vi "ConfigPlots.vi"(5 "曲线自定义封存数组":refnum<vi>, 7 "Y轴手配":refnum<vi>, 8 "Y标尺总数":i32, 9 "曲线手配":refnum<vi>, 10 "已选信号列表":refnum<vi>) -> ()   [LabVIEW 2015]
uses:
  Ctrls/btnSeeOrNot.ctl
panel:
  out "txtYlink":string
  out "txtUnit":string
  out "txtCurves":string
  out "txtYVisable":string
  out "txtSignal":string
  out "txtRename":string
  out "txtYName":string
  out "txtYsn":string
  out "txtYSetupTitle":string caption="txtYSetup"
  out "txtCurvesSetup":string
  in  "取消并退出按钮":bool
  in  "保存曲线设置按钮":bool
  in  "曲线设置输入簇数组":T1(array[cluster]) {"关联Y轴" min=1 max=8 format="Y轴%d"; "曲线序号" format="曲线%d"}
  in  "曲线簇":T2={"曲线序号"=0, "SignalName"="", "SignalTag"="", "自定义名"="", "单位"="", "关联Y轴"=1} {"关联Y轴" min=1 max=8 format="Y轴%d"; "曲线序号" format="曲线%d"}
  in  "Y簇":T4
  in  "Y轴配置":T5(array[cluster])
  out "自动Y轴配置":cluster{"Y轴序号":u8, "Y轴名称":string, "可见性":bool}[](array[cluster])
  out "自动曲线配置":T1(array[cluster])
  in  "曲线配置簇":T2
  in  "Y轴配置簇":cluster{"Y轴序号":u8, "Y轴名称":string, "可见性":bool}
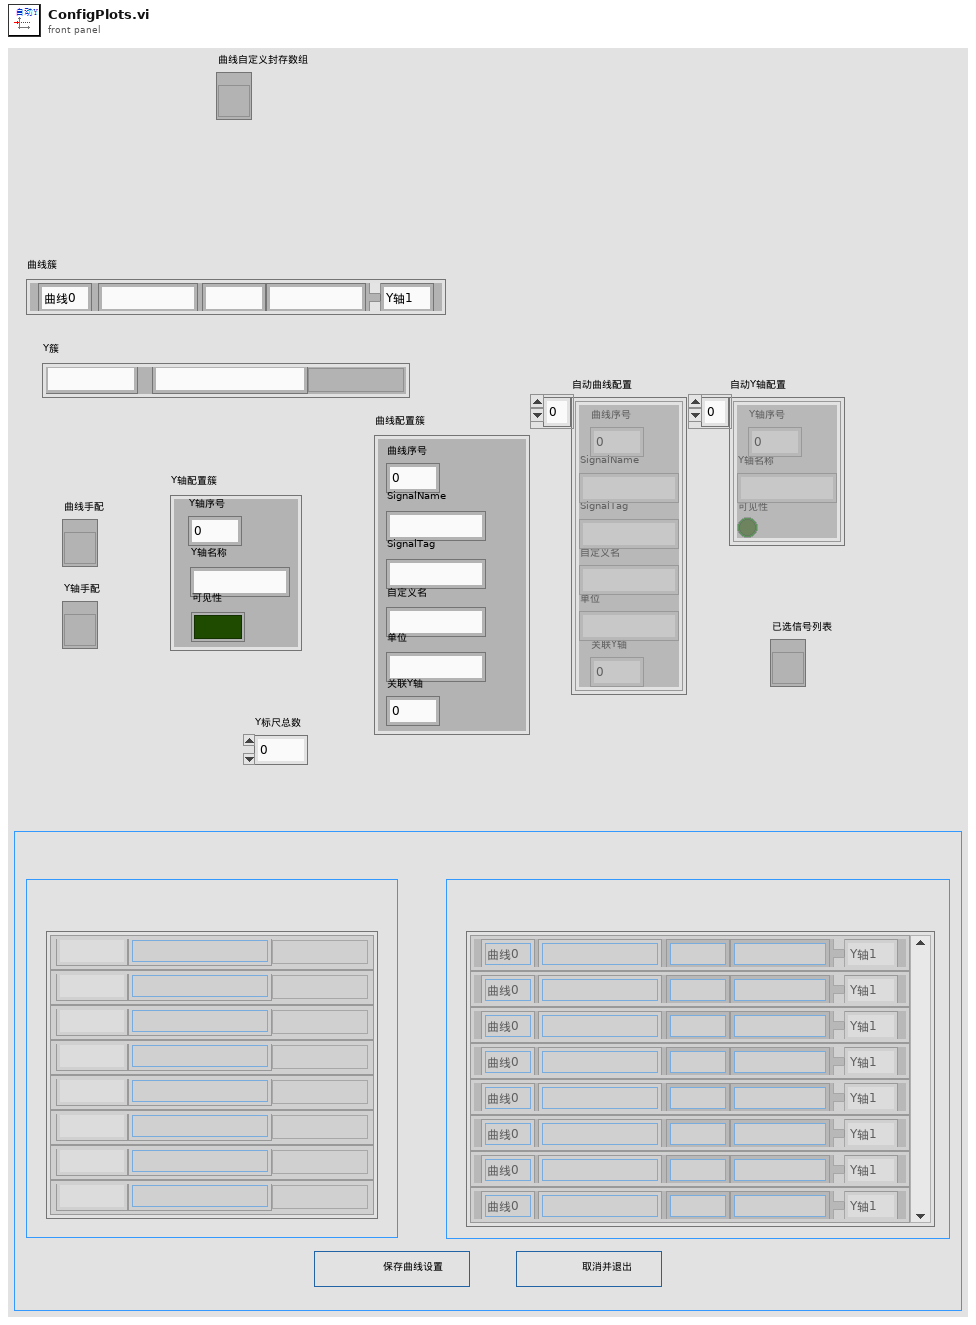
[diagram p1: front panel]
types:
  T1 = cluster{"曲线序号":u8, "SignalName":string, "SignalTag":string, "自定义名":string, "单位":string, "关联Y轴":u8}[]
  T2 = cluster{"曲线序号":u8, "SignalName":string, "SignalTag":string, "自定义名":string, "单位":string, "关联Y轴":u8}
  T3 = typedef "btnSeeOrNot.ctl" = bool
  T4 = cluster{"Y轴名称 2":string, "Y轴序号 2":string, "可见性":T3}
  T5 = cluster{"Y轴名称 2":string, "Y轴序号 2":string, "可见性":T3}[]
  T6 = typedef "可不可见.ctl" = bool
  T7 = cluster{"Y轴名称 2":string, "Y轴序号 2":string, "可见性":T6}
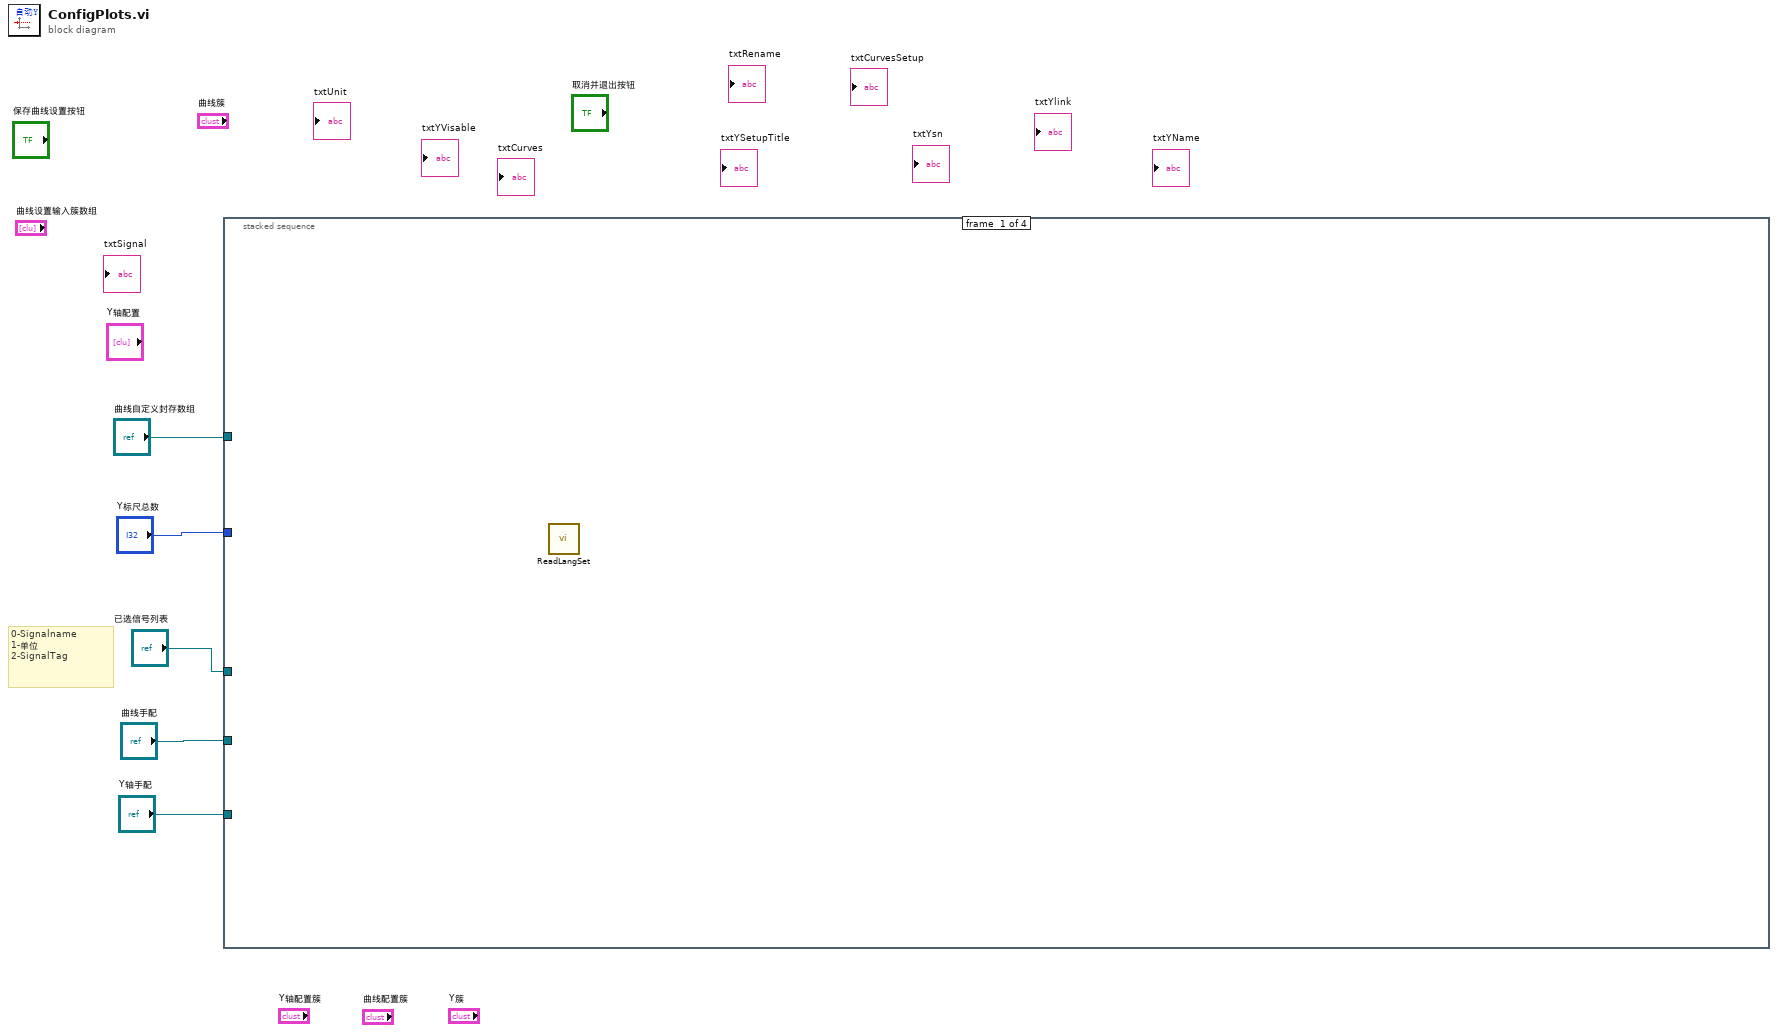
[diagram p0: block diagram]
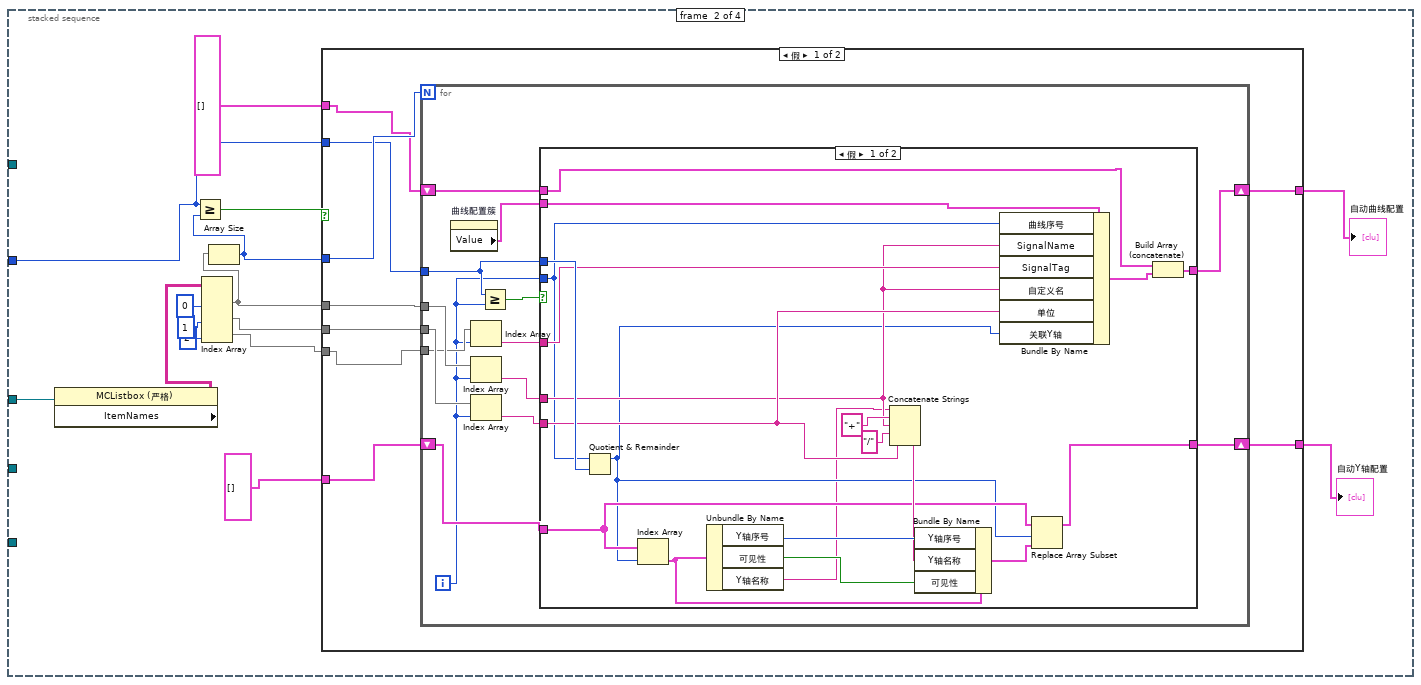
[diagram p2: hidden frame]
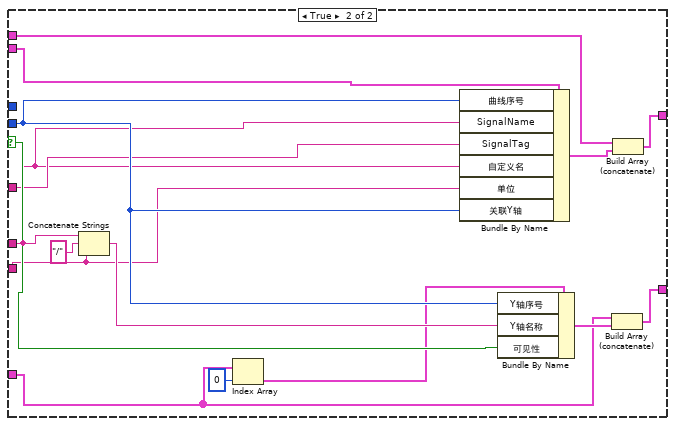
[diagram p3: hidden frame]
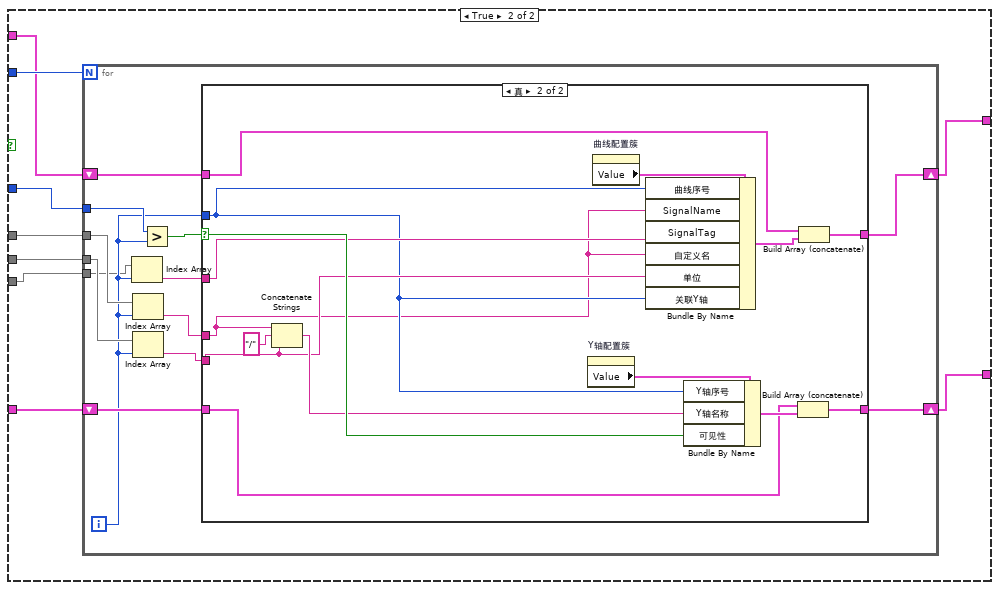
[diagram p4: hidden frame]
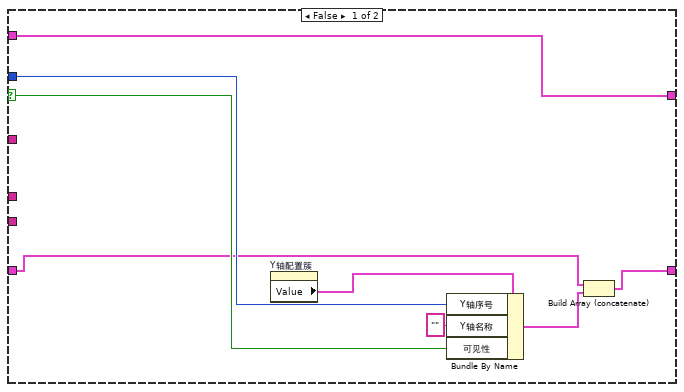
[diagram p5: hidden frame]
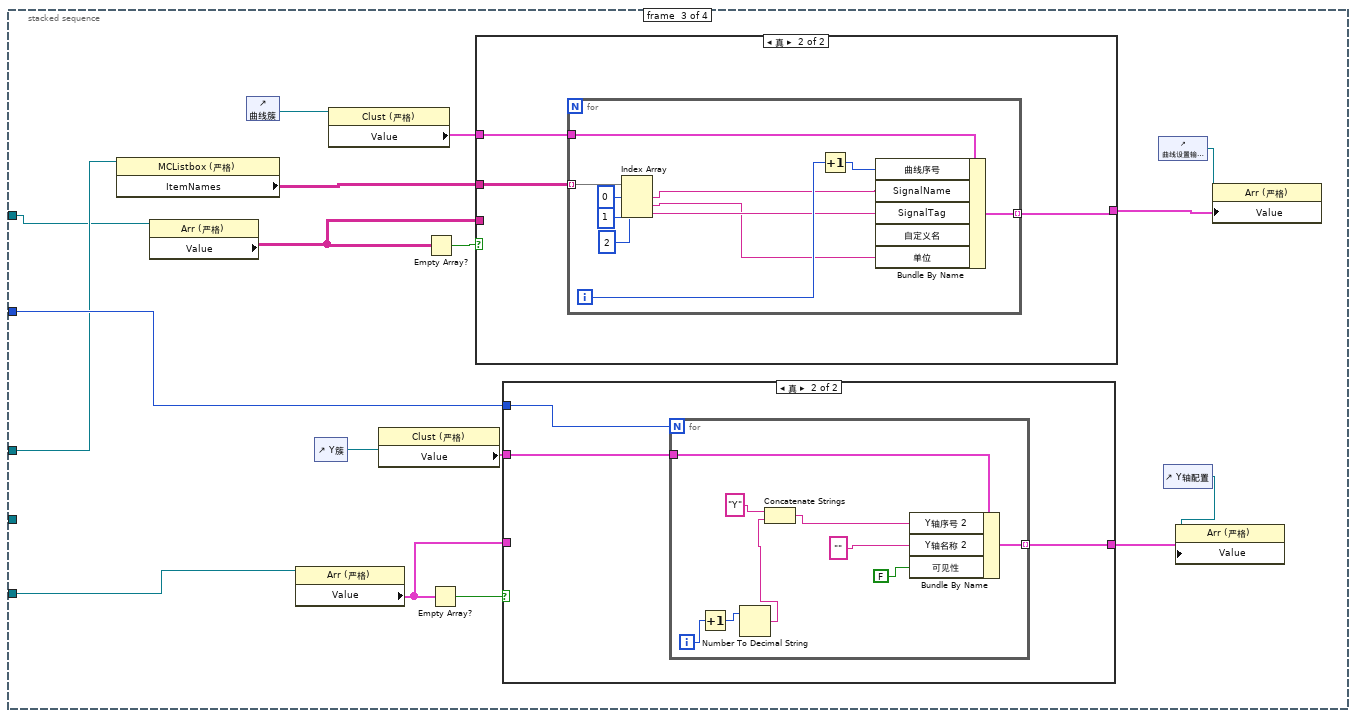
[diagram p6: hidden frame]
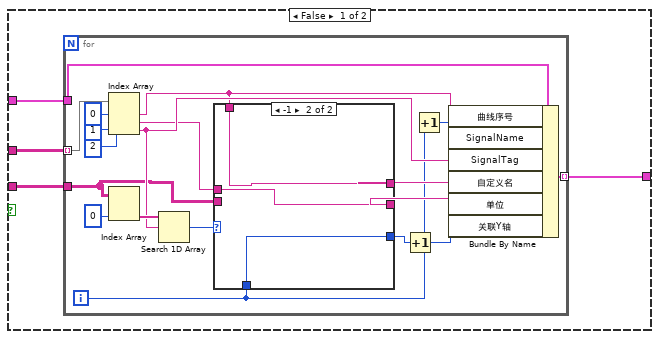
[diagram p7: hidden frame]
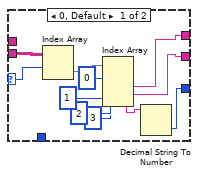
[diagram p8: hidden frame]
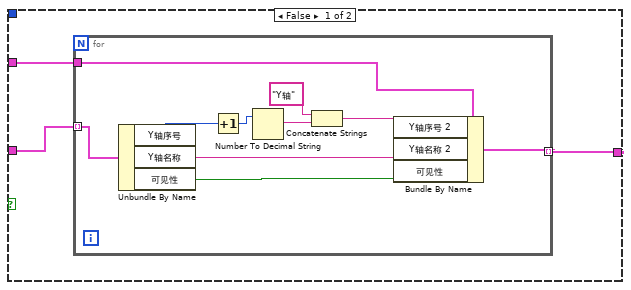
[diagram p9: hidden frame]
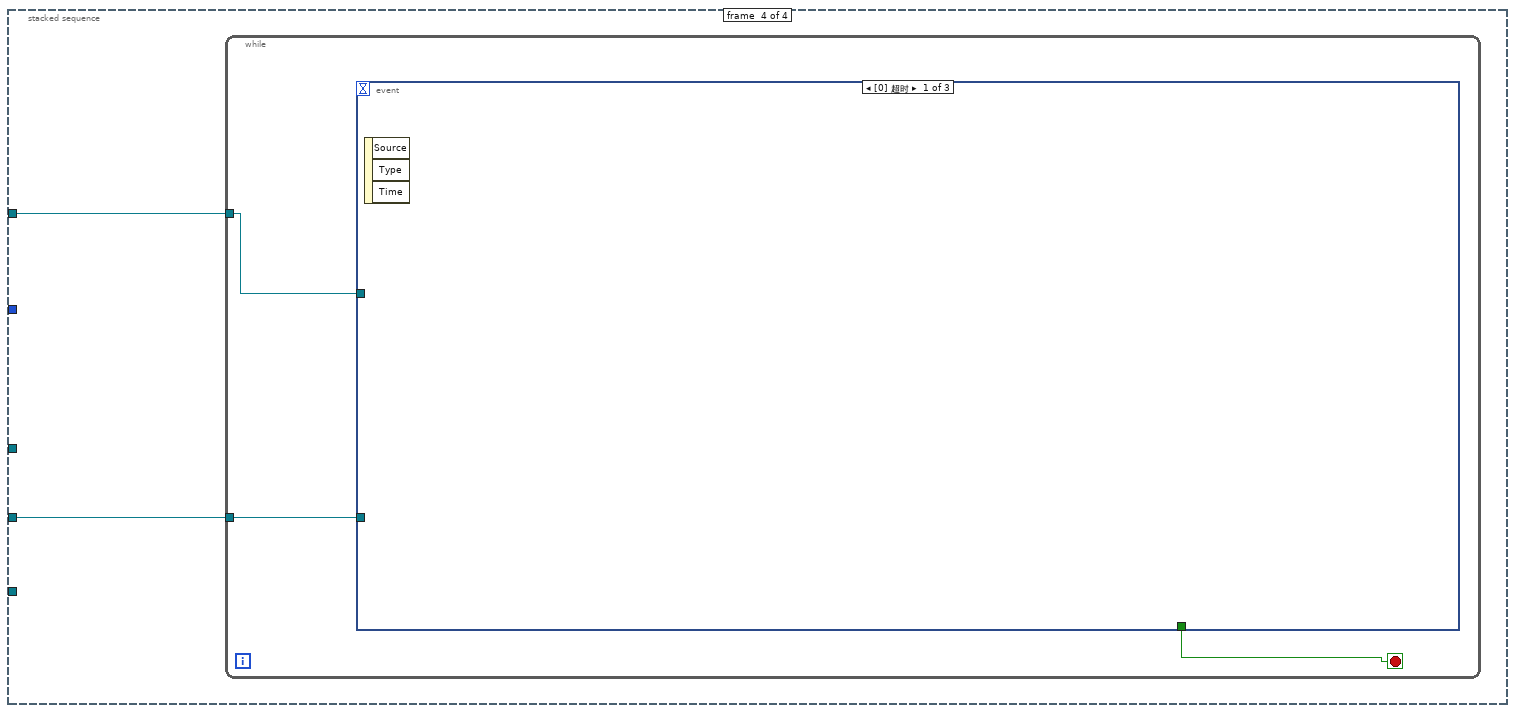
[diagram p10: hidden frame]
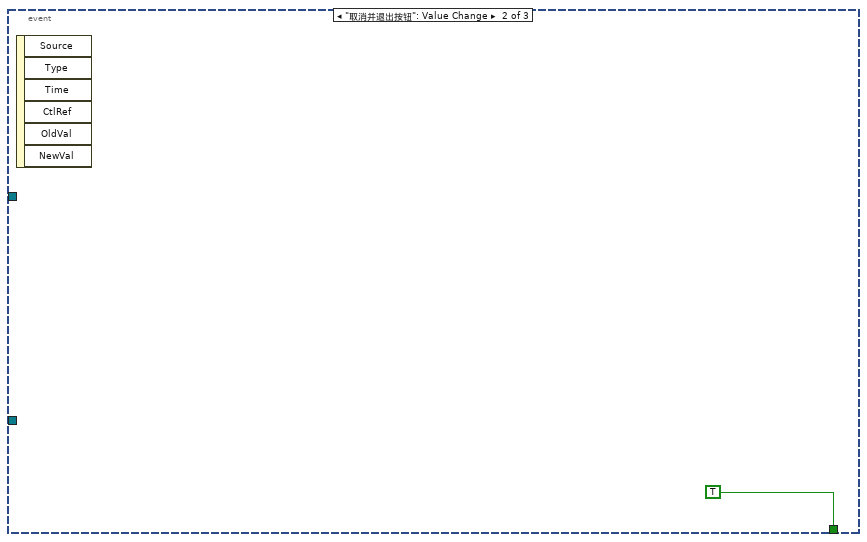
[diagram p11: hidden frame]
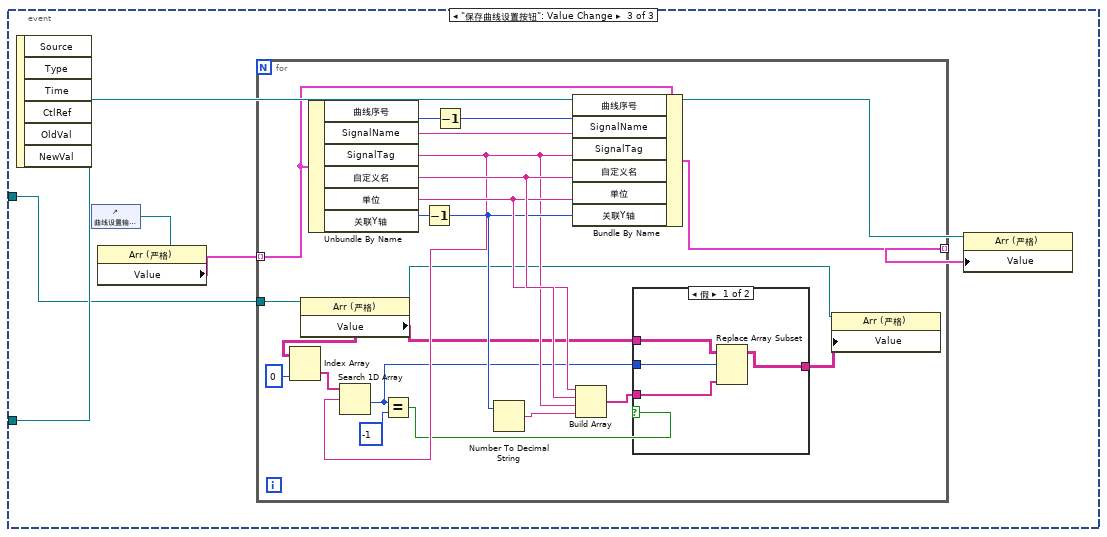
[diagram p12: hidden frame]
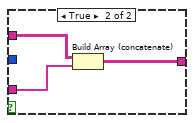
[diagram p13: hidden frame]
diagram:
  # "0-Signalname\n1-单位\n2-SignalTag"
  n1 = stacked-sequence {
    tunnel: "Y标尺总数" -> [_ w16 w134 _]
    tunnel: "已选信号列表" -> [_ w7 w127 _]
    tunnel: "曲线手配" -> [_ _ _ w219]
    tunnel: "Y轴手配" -> [_ _ w141 _]
    tunnel: "曲线自定义封存数组" -> [_ _ w125 w218]
    frame #0 {
      n2 = call "ReadLangSet.vi"() -> ()  [unwired: 11 in, 1 out]
    }
    frame #1 {
      n3 = property class="MCListbox (严格)"(reference=w7) -> ("ItemNames"=w6:string[][])  [unwired: 1 in, 2 out]
      n4 = Index Array(array=w6, index (col) #1=0 ("禁用的索引 (列)"), index (col) #2=1 ("索引 (列)"), index (col) #3=2 ("索引 (列)")) -> (element #1=w18:string[], element #2=w19:string[], element #3=w12:string[])  [unwired: 3 in]
      n5 = Array Size(array=w18) -> (size(s)=w20:i32)
      n6 = Greater Or Equal?(x=w16, y=w20) -> (x >= y?=w15:bool)
      n7 = case shown="假" w15 {
        tunnel: w16 -> [w26 w88]
        tunnel: w18 -> [w28 w87]
        tunnel: w19 -> [w29 w86]
        tunnel: w20 -> [w27 w85]
        tunnel: w12 -> [w24 w84]
        tunnel: cluster{"Y轴序号":u8, "Y轴名称":string, "可见性":bool}[] [] -> [w25 w83]
        tunnel: T1 [] -> [w23 w82]
        tunnel: [w22 w80] -> w8
        tunnel: [w21 w81] -> w9
        frame False {
          n8 = for {
            N: w27 -> [_]
            tunnel: w28 -> [w40]
            tunnel: w29 -> [w39]
            tunnel: w26 -> [w38]
            shift-right: [w37] -> w22
            shift-left: w25 -> [w36]
            tunnel: w24 -> [w35]
            shift-right: [w32] -> w21
            shift-left: w23 -> [w31]
            i -> [w34]
            n9 = property on="曲线配置簇" class="Clust (严格)"() -> ("Value"=w30:T2)  [unwired: 2 in, 2 out]
            n10 = Index Array(array=w35, index=w34) -> (element=w33:string)
            n11 = Index Array(array=w40, index=w34) -> (element=w42:string)
            n12 = Index Array(array=w39, index=w34) -> (element=w41:string)
            n13 = Greater Or Equal?(x=w38, y=w34) -> (x >= y?=w43:bool)
            n14 = case shown="假" w43 {
              selector: w43 -> [_ w75]
              tunnel: w34 -> [w56 w73]
              tunnel: w42 -> [w57 w70]
              tunnel: w41 -> [w59 w72]
              tunnel: w38 -> [w63 _]
              tunnel: [w46 w76] -> w37
              tunnel: w36 -> [w49 w67]
              tunnel: w33 -> [w58 w71]
              tunnel: [w54 w69] -> w32
              tunnel: w31 -> [w55 w68]
              tunnel: w30 -> [w44 w64]
              frame False {
                n15 = Quotient & Remainder(x=w56, y=w63) -> (x-y*floor(x/y)=w48:i32)  [unwired: 1 out]
                n16 = Index Array(array=w49, index=w48) -> (element=w53:cluster{"Y轴序号":u8, "Y轴名称":string, "可见性":bool})
                n17 = Unbundle By Name(w53) -> ("Y轴序号"=w52:u8, "可见性"=w50:bool, "Y轴名称"=w45:string)
                n18 = Concatenate Strings(w45, "+" ("字符串"), w57, "/" ("字符串"), w59) -> (w51:string)
                n19 = Bundle By Name(cluster=w53, "Y轴序号"=w52, "Y轴名称"=w51, "可见性"=w50) -> (w47:cluster{"Y轴序号":u8, "Y轴名称":string, "可见性":bool})
                n20 = Bundle By Name(cluster=w44, "曲线序号"=w56, "SignalName"=w57, "SignalTag"=w58, "自定义名"=w57, "单位"=w59, "关联Y轴"=w48) -> (w60:T2)
                n21 = Replace Array Subset(array=w49, new element=w47, index=w48) -> (w46:cluster{"Y轴序号":u8, "Y轴名称":string, "可见性":bool}[])
                n22 = Build Array (concatenate)(w55, w60) -> (w54:T1)
              }
              frame True {
                n23 = Concatenate Strings(w70, "/" ("字符串"), w72) -> (w74:string)
                n24 = Index Array(array=w67, index=0 ("索引")) -> (element=w65:cluster{"Y轴序号":u8, "Y轴名称":string, "可见性":bool})
                n25 = Bundle By Name(cluster=w64, "曲线序号"=w73, "SignalName"=w70, "SignalTag"=w71, "自定义名"=w70, "单位"=w72, "关联Y轴"=w73) -> (w77:T2)
                n26 = Bundle By Name(cluster=w65, "Y轴序号"=w73, "Y轴名称"=w74, "可见性"=w75) -> (w78:cluster{"Y轴序号":u8, "Y轴名称":string, "可见性":bool})
                n27 = Build Array (concatenate)(w67, w78) -> (w76:cluster{"Y轴序号":u8, "Y轴名称":string, "可见性":bool}[])
                n28 = Build Array (concatenate)(w68, w77) -> (w69:T1)
              }
            }
          }
        }
        frame True {
          n29 = for {
            N: w88 -> [_]
            tunnel: w87 -> [w98]
            tunnel: w86 -> [w97]
            tunnel: w85 -> [w96]
            shift-right: [w95] -> w80
            shift-left: w83 -> [w94]
            tunnel: w84 -> [w92]
            shift-right: [w90] -> w81
            shift-left: w82 -> [w89]
            i -> [w93]
            n30 = Index Array(array=w92, index=w93) -> (element=w91:string)
            n31 = Index Array(array=w98, index=w93) -> (element=w100:string)
            n32 = Index Array(array=w97, index=w93) -> (element=w99:string)
            n33 = Greater?(x=w96, y=w93) -> (0:w101:bool)
            n34 = case shown="真" w101 {
              selector: w101 -> [w107 w122]
              tunnel: w93 -> [w108 w114]
              tunnel: w100 -> [_ w110]
              tunnel: w99 -> [_ w116]
              tunnel: [w106 w119] -> w95
              tunnel: w94 -> [w104 w118]
              tunnel: w91 -> [_ w115]
              tunnel: [w103 w112] -> w90
              tunnel: w89 -> [w103 w111]
              frame False {
                n35 = property on="Y轴配置簇" class="Clust (严格)"() -> ("Value"=w102:cluster{"Y轴序号":u8, "Y轴名称":string, "可见性":bool})  [unwired: 2 in, 2 out]
                n36 = Bundle By Name(cluster=w102, "Y轴序号"=w108, "Y轴名称"="", "可见性"=w107) -> (w105:cluster{"Y轴序号":u8, "Y轴名称":string, "可见性":bool})
                n37 = Build Array (concatenate)(w104, w105) -> (w106:cluster{"Y轴序号":u8, "Y轴名称":string, "可见性":bool}[])
              }
              frame True {
                n38 = Concatenate Strings(w110, "/" ("字符串"), w116) -> (w121:string)
                n39 = property on="Y轴配置簇" class="Clust (严格)"() -> ("Value"=w123:cluster{"Y轴序号":u8, "Y轴名称":string, "可见性":bool})  [unwired: 2 in, 2 out]
                n40 = property on="曲线配置簇" class="Clust (严格)"() -> ("Value"=w117:T2)  [unwired: 2 in, 2 out]
                n41 = Bundle By Name(cluster=w117, "曲线序号"=w114, "SignalName"=w110, "SignalTag"=w115, "自定义名"=w110, "单位"=w116, "关联Y轴"=w114) -> (w113:T2)
                n42 = Bundle By Name(cluster=w123, "Y轴序号"=w114, "Y轴名称"=w121, "可见性"=w122) -> (w120:cluster{"Y轴序号":u8, "Y轴名称":string, "可见性":bool})
                n43 = Build Array (concatenate)(w118, w120) -> (w119:cluster{"Y轴序号":u8, "Y轴名称":string, "可见性":bool}[])
                n44 = Build Array (concatenate)(w111, w113) -> (w112:T1)
              }
            }
          }
        }
      }
      "自动Y轴配置" <- w8
      "自动曲线配置" <- w9
    }
    frame #2 {
      n45 = property class="MCListbox (严格)"(reference=w127) -> ("ItemNames"=w126:string[][])  [unwired: 1 in, 2 out]
      n46 = property class="Arr (严格)"(reference=w125) -> ("Value"=w128:string[][])  [unwired: 1 in, 2 out]
      n47 = control-ref of="曲线簇"() -> (w131:refnum<vi>)
      n48 = property class="Arr (严格)"(reference=w141) -> ("Value"=w139:cluster{"Y轴序号":u8, "Y轴名称":string, "可见性":bool}[])  [unwired: 1 in, 2 out]
      n49 = control-ref of="Y簇"() -> (w136:refnum<vi>)
      n50 = property class="Clust (严格)"(reference=w131) -> ("Value"=w130:T2)  [unwired: 1 in, 2 out]
      n51 = property class="Clust (严格)"(reference=w136) -> ("Value"=w135:T7)  [unwired: 1 in, 2 out]
      n52 = Empty Array?(array=w128) -> (empty?=w133:bool)
      n53 = Empty Array?(array=w139) -> (empty?=w140:bool)
      n54 = case shown="真" w133 {
        tunnel: w130 -> [w145 w180]
        tunnel: [w144 w179] -> w129
        tunnel: w128 -> [w143 _]
        tunnel: w126 -> [w142 w181]
        frame False {
          n55 = for {
            tunnel: w145 -> [w164]
            tunnel: [w163] -> w144 mode=indexing
            tunnel: w143 -> [w148]
            tunnel: w142 -> [w161] mode=indexing
            i -> [w149]
            n56 = Index Array(array=w161, index #1=0 ("索引"), index #2=1 ("索引"), index #3=2 ("索引")) -> (element #1=w150:string, element #2=w152:string, element #3=w155:string)
            n57 = Index Array(array=w148, index (col)=0 ("禁用的索引 (列)")) -> (element=w156:string[])  [unwired: 1 in]
            n58 = Search 1D Array(1D array=w156, element=w155) -> (index of element=w154:i32)  [unwired: 1 in]
            n59 = case shown="-1" w154 {
              selector: w154 -> [w174 _]
              tunnel: [w167 w178] -> w153
              tunnel: w152 -> [_ w178]
              tunnel: [w168 w177] -> w151
              tunnel: w150 -> [_ w177]
              tunnel: w149 -> [_ w176]
              tunnel: w148 -> [w175 _]
              tunnel: [w165 w176] -> w146
              frame 0, Default {
                n60 = Index Array(array=w175, index (row)=w174) -> (element=w173:string[])  [unwired: 1 in]
                n61 = Index Array(array=w173, index #1=0 ("索引"), index #2=1 ("索引"), index #3=2 ("索引"), index #4=3 ("索引")) -> (element #2=w168:string, element #3=w167:string, element #4=w166:string)  [unwired: 1 out]
                n62 = Decimal String To Number(string=w166) -> (number=w165:i32)  [unwired: 2 in, 1 out]
              }
              frame -1 {
              }
            }
            n63 = Increment(x=w146) -> (x+1=w147:i32)
            n64 = Increment(x=w149) -> (x+1=w162:i32)
            n65 = Bundle By Name(cluster=w164, "曲线序号"=w162, "SignalName"=w150, "SignalTag"=w155, "自定义名"=w151, "单位"=w153, "关联Y轴"=w147) -> (w163:T2)
          }
        }
        frame True {
          n66 = for {
            tunnel: w181 -> [w189] mode=indexing
            tunnel: w180 -> [w192]
            tunnel: [w182] -> w179 mode=indexing
            i -> [w191]
            n67 = Index Array(array=w189, index #1=0 ("索引"), index #2=1 ("索引"), index #3=2 ("索引")) -> (element #1=w184:string, element #2=w183:string, element #3=w185:string)
            n68 = Increment(x=w191) -> (x+1=w190:i32)
            n69 = Bundle By Name(cluster=w192, "曲线序号"=w190, "SignalName"=w184, "SignalTag"=w185, "自定义名"=w184, "单位"=w183) -> (w182:T2)
          }
        }
      }
      n70 = case shown="真" w140 {
        tunnel: w139 -> [w195 _]
        tunnel: [w194 w206] -> w137
        tunnel: w135 -> [w193 w207]
        tunnel: w134 -> [_ w208]
        frame False {
          n71 = for {
            tunnel: w195 -> [w205] mode=indexing
            tunnel: [w197] -> w194 mode=indexing
            tunnel: w193 -> [w196]
            n72 = Unbundle By Name(w205) -> ("Y轴序号"=w204:u8, "Y轴名称"=w199:string, "可见性"=w200:bool)
            n73 = Increment(x=w204) -> (x+1=w203:u8)
            n74 = Number To Decimal String(number=w203) -> (decimal integer string=w202:string)  [unwired: 1 in]
            n75 = Concatenate Strings("Y轴" ("字符串"), w202) -> (w198:string)
            n76 = Bundle By Name(cluster=w196, "Y轴序号 2"=w198, "Y轴名称 2"=w199, "可见性"=w200) -> (w197:T7)
          }
        }
        frame True {
          n77 = for {
            N: w208 -> [_]
            tunnel: w207 -> [w217]
            tunnel: [w216] -> w206 mode=indexing
            i -> [w215]
            n78 = Increment(x=w215) -> (x+1=w212:i32)
            n79 = Number To Decimal String(number=w212) -> (decimal integer string=w211:string)  [unwired: 1 in]
            n80 = Concatenate Strings("Y" ("字符串"), w211) -> (w209:string)
            n81 = Bundle By Name(cluster=w217, "Y轴序号 2"=w209, "Y轴名称 2"="", "可见性"=FALSE) -> (w216:T7)
          }
        }
      }
      n82 = control-ref of="曲线设置输入簇数组"() -> (w132:refnum<vi>)
      n83 = control-ref of="Y轴配置"() -> (w138:refnum<vi>)
      n84 = property class="Arr (严格)"(reference=w138, "Value"=w137) -> ()  [unwired: 1 in, 2 out]
      n85 = property class="Arr (严格)"(reference=w132, "Value"=w129) -> ()  [unwired: 1 in, 2 out]
    }
    frame #3 {
      n86 = while {
        tunnel: w219 -> [w221]
        tunnel: w218 -> [w220]
        stop <- w222 stop-if-true
        n87 = event shown="[0] 超时" {
          selector: _ -> [_ _ _]
          dyn-events: _ -> [_ _ _]
          timeout: _ -> [_ _ _]
          tunnel: [_ TRUE _] -> w222
          tunnel: w221 -> [_ _ w225]
          tunnel: w220 -> [_ _ w224]
          event Timeout {
            n88 = event-data() -> ()  [unwired: 1 in, 3 out]
          }
          event "取消并退出按钮": Value Change {
            n89 = event-data() -> ()  [unwired: 1 in, 6 out]
          }
          event "保存曲线设置按钮": Value Change {
            n90 = event-data() -> ()  [unwired: 1 in, 6 out]
            n91 = control-ref of="曲线设置输入簇数组"() -> (w228:refnum<vi>)
            n92 = property class="Arr (严格)"(reference=w228) -> ("Value"=w227:T1)  [unwired: 1 in, 2 out]
            n93 = for {
              tunnel: w227 -> [w247] mode=indexing
              tunnel: [w244] -> w226 mode=indexing
              tunnel: w224 -> [w236]
              n94 = property class="Arr (严格)"(reference=w236) -> (reference out=w234:refnum<vi>, "Value"=w235:string[][])  [unwired: 1 in, 1 out]
              n95 = Index Array(array=w235, index (col)=0 ("禁用的索引 (列)")) -> (element=w237:string[])  [unwired: 1 in]
              n96 = Unbundle By Name(w247) -> ("曲线序号"=w248:u8, "SignalName"=w245:string, "SignalTag"=w240:string, "自定义名"=w243:string, "单位"=w242:string, "关联Y轴"=w249:u8)
              n97 = Search 1D Array(1D array=w237, element=w240) -> (index of element=w229:i32)  [unwired: 1 in]
              n98 = Equal?(x=w229, y=-1) -> (x = y?=w230:bool)
              n99 = Decrement(x=w249) -> (x-1=w241:u8)
              n100 = Decrement(x=w248) -> (x-1=w246:u8)
              n101 = Number To Decimal String(number=w241) -> (decimal integer string=w232:string)  [unwired: 1 in]
              n102 = Bundle By Name(cluster=w247, "曲线序号"=w246, "SignalName"=w245, "SignalTag"=w240, "自定义名"=w243, "单位"=w242, "关联Y轴"=w241) -> (w244:T2)
              n103 = Build Array(w240, w243, w242, w232) -> (w231:string[])
              n104 = case shown="假" w230 {
                tunnel: w235 -> [w253 w256]
                tunnel: [w250 w255] -> w233
                tunnel: w231 -> [w252 w254]
                tunnel: w229 -> [w251 _]
                frame False {
                  n105 = Replace Array Subset(array=w253, new element=w252, index (row)=w251) -> (w250:string[][])  [unwired: 1 in]
                }
                frame True {
                  n106 = Build Array (concatenate)(w256, w254) -> (w255:string[][])
                }
              }
              n107 = property class="Arr (严格)"(reference=w234, "Value"=w233) -> ()  [unwired: 1 in, 2 out]
            }
            n108 = property class="Arr (严格)"(reference=w225, "Value"=w226) -> ()  [unwired: 1 in, 2 out]
          }
        }
      }
    }
  }
